vi "Calculate Next Parameter.vi"(8 "error in (no error)":errorcluster, 10 "first?":bool, 11 "SimpleExperimentService in":refnum<class "SimpleExperimentService.lvclass">) -> (0 "error out":errorcluster, 1 "Stop?":bool, 2 "Parameter":dbl, 3 "SimpleExperimentService out":refnum<class "SimpleExperimentService.lvclass">)   [LabVIEW 2014, in "SimpleExperimentService.lvclass"]
uses:
  SimpleExperimentService.lvclass
  SimpleExperimentService.lvclass/SimpleExperimentService.ctl
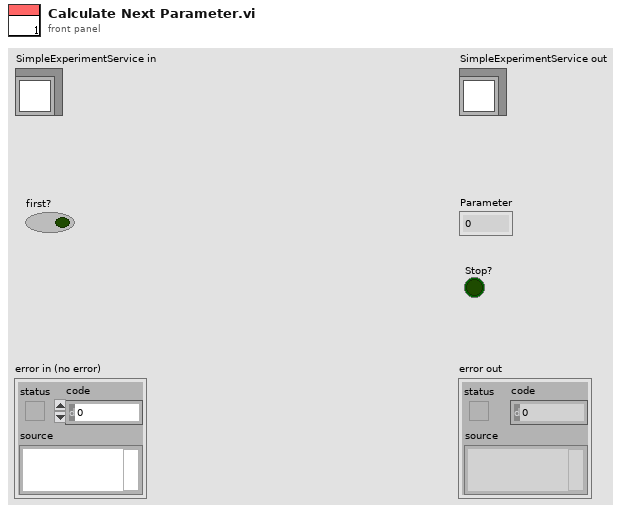
[diagram p1: front panel]
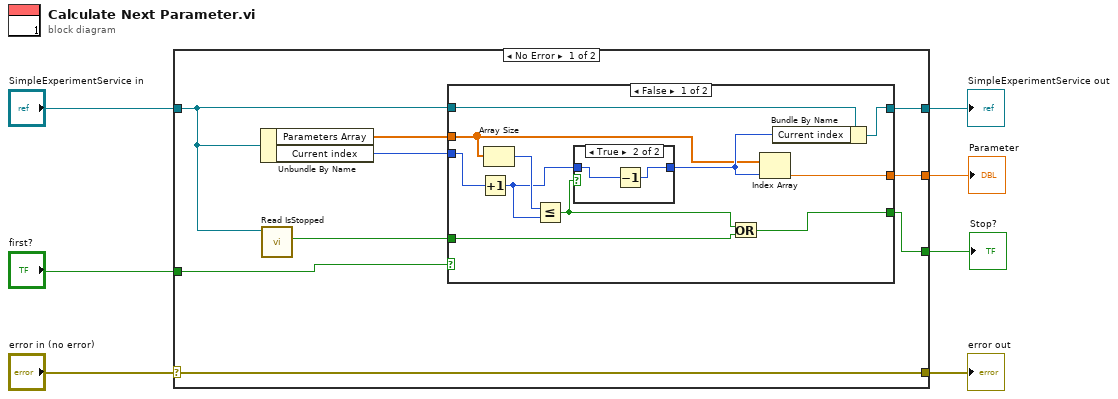
[diagram p0: block diagram]
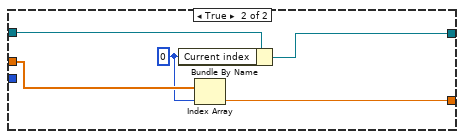
[diagram p3: hidden frame]
diagram:
  n1 = case shown="No Error" "error in (no error)" {
    selector: "error in (no error)" -> [w11 w37]
    tunnel: [w11 w37] -> w6
    tunnel: [w10 w36] -> w4
    tunnel: "SimpleExperimentService in" -> [w9 w36]
    tunnel: "first?" -> [w14 _]
    tunnel: [w13 _] -> w2
    tunnel: [w12 _] -> w1
    frame No Error {
      n2 = Unbundle By Name(w9) -> ("Parameters Array"=w15:dbl[], "Current index"=w16:u32)
      n3 = call-dynamic "Read IsStopped.vi"("ExperimentService in"=w9) -> ("IsStopped"=w8:bool)  [unwired: 8 in, 2 out]
      n4 = case shown="False" w14 {
        tunnel: w9 -> [w24 w35]
        tunnel: w15 -> [w20 w33]
        tunnel: w16 -> [w27 _]
        tunnel: [w22 w32] -> w13
        tunnel: [w18 _] -> w12
        tunnel: [w23 w34] -> w10
        tunnel: w8 -> [w17 _]
        frame False {
          n5 = Increment(x=w27) -> (x+1=w25:u32)
          n6 = Array Size(array=w20) -> (size(s)=w26:i32)
          n7 = Less Or Equal?(x=w26, y=w25) -> (x <= y?=w19:bool)
          n8 = case shown="True" w19 {
            tunnel: w25 -> [w28 w30]
            tunnel: [w28 w29] -> w21
            frame False {
            }
            frame True {
              n9 = Decrement(x=w30) -> (x-1=w29:u32)
            }
          }
          n10 = Or(x=w19, y=w17) -> (x .or. y?=w18:bool)
          n11 = Index Array(array=w20, index=w21) -> (element=w22:dbl)
          n12 = Bundle By Name(cluster=w24, "Current index"=w21) -> (w23:refnum<class "SimpleExperimentService.lvclass">)
        }
        frame True {
          w31 = u32 0 ("Current index")
          n13 = Bundle By Name(cluster=w35, "Current index"=w31) -> (w34:refnum<class "SimpleExperimentService.lvclass">)
          n14 = Index Array(array=w33, index=w31) -> (element=w32:dbl)
        }
      }
    }
    frame Error {
    }
  }
  "error out" <- w6
  "SimpleExperimentService out" <- w4
  "Parameter" <- w2
  "Stop?" <- w1
